vi "AG364x Voltage Controler.vi"(8 "error in (no error)":errorcluster, 9 "Select CH":string[](array[string]), 10 "VDD/VIO":dbl[](array[numeric]), 11 "VISA In":refnum<visa-resource-name>) -> (0 "error out":errorcluster, 3 "VISA Out":refnum<visa-resource-name>)   [LabVIEW 2017]
uses:
  Test Equipment/E364x/Agilent E364X Series/Agilent E364X Series.lvlib
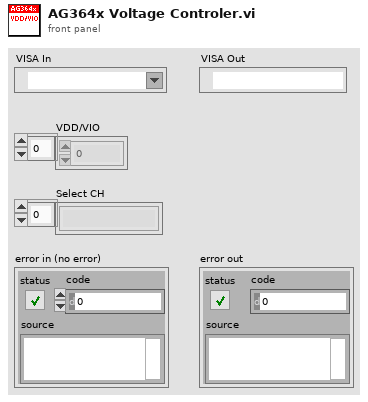
[diagram p1: front panel]
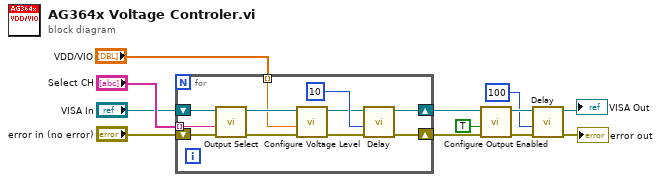
[diagram p0: block diagram]
diagram:
  n1 = for {
    shift-right: [w21] -> w4
    shift-left: "error in (no error)" -> [w20]
    shift-right: [w12] -> w5
    shift-left: "VISA In" -> [w19]
    tunnel: "Select CH" -> [w15] mode=indexing
    tunnel: "VDD/VIO" -> [w14] mode=indexing
    n2 = call "Output Select.vi"("error in (no error)"=w20, "Instrument Select (Output 1)"=w15, "VISA resource name"=w19) -> ("error out"=w18:errorcluster, "VISA resource name out"=w17:refnum<visa-resource-name>)  [unwired: 7 in]
    n3 = call "Configure Voltage Level.vi"("error in (no error)"=w18, "Level (0.0 Volts)"=w14, "VISA resource name"=w17) -> ("error out"=w13:errorcluster, "VISA resource name out"=w12:refnum<visa-resource-name>)  [unwired: 7 in]
    n4 = call "Delay.vi"("error in (no error)"=w13, "Delay"=u32 10) -> ("error out"=w21:errorcluster)  [unwired: 9 in]
  }
  n5 = call "Configure Output Enabled.vi"("error in (no error)"=w4, "Output Enabled (F: Off)"=TRUE, "VISA resource name"=w5) -> ("error out"=w3:errorcluster, "VISA resource name out"=→"VISA Out":refnum<visa-resource-name>)  [unwired: 7 in]
  n6 = call "Delay.vi"("error in (no error)"=w3, "Delay"=u32 100) -> ("error out"=→"error out":errorcluster)  [unwired: 9 in]
